vi "Read Sweep Configuration Example.vi"   [LabVIEW 2019, in "Sweep Control.lvclass"]
uses:
  Sweep Control.lvclass
  Typedefs/Enum - Experiments.ctl
  Typedefs/Continuous B Sweep JSON--Cluster.ctl
  Typedefs/Enum - Priority.ctl
  Typedefs/Enum - Action.ctl
  Typedefs/Cluster - ScanControl.ctl
  Typedefs/ScanControl.ctl
  Typedefs/Cluster - ScanParamters.ctl
  Typedefs/ScanParamters.ctl
  Typedefs/Sweep Control JSON--Cluster.ctl
  <userlib>/LevyLab/Transport/Transport/Typedefs/Lockin_Sweep JSON--Cluster.ctl
  <userlib>/LevyLab/Transport/Transport/Transport.lvclass
  <userlib>/LevyLab/Transport/Control Experiment/Typedefs/Wiring Description--cluster.ctl
  <userlib>/LevyLab/Transport/Control Experiment/Control Experiment.lvclass
  <userlib>/LevyLab/Transport/Control Experiment/Typedefs/Experiment Description--cluster.ctl
  <userlib>/LevyLab/Lockin-Multichannel/Instrument.DAQ/Typedefs/REF.Channel--Cluster--Array.ctl
  <userlib>/LevyLab/Lockin-Multichannel/Instrument.DAQ/Instrument.DAQ.lvclass
  <userlib>/LevyLab/Lockin-Multichannel/Instrument.DAQ/Typedefs/AO.Channel--Cluster--Array.ctl
  <userlib>/LevyLab/Transport/Control Experiment/Typedefs/Instruments--cluster.ctl
  <userlib>/LevyLab/Krohn Hite 7008/KH7008/typedefs/Filter--Enum.ctl
  <userlib>/LevyLab/Krohn Hite 7008/KH7008/KH7008.lvlib
  <userlib>/LevyLab/Krohn Hite 7008/KH7008/typedefs/couple--Enum.ctl
  <userlib>/LevyLab/Krohn Hite 7008/KH7008/typedefs/shunt--enum.ctl
  <userlib>/LevyLab/Krohn Hite 7008/KH7008/typedefs/Input--Enum.ctl
  <userlib>/LevyLab/Krohn Hite 7008/KH7008/typedefs/gain--enum.ctl
  <userlib>/LevyLab/Krohn Hite 7008/KH7008/typedefs/channel--numeric.ctl
  <userlib>/LevyLab/Krohn Hite 7008/KH7008/typedefs/channelProperties--Cluster.ctl
  <userlib>/LevyLab/Krohn Hite 7008/KH7008/typedefs/allChannelProperties--Array.ctl
  <userlib>/LevyLab/Lockin-Multichannel/Instrument.DAQ/Typedefs/AO.Channel.Function--Enum.ctl
  <userlib>/LevyLab/Lockin-Multichannel/Instrument.DAQ/Typedefs/AO.Channel--Cluster.ctl
  <userlib>/LevyLab/Lockin-Multichannel/Instrument.DAQ/Typedefs/REF.Channel--Cluster.ctl
  <userlib>/LevyLab/Transport/Control Experiment/Typedefs/Instrument Types--enum.ctl
panel:
  # "See block diagram for example of how to use ReadSweepConfigurationFile.vi"
types:
  T1 = typedef "Transport.lvclass/Lockin_Sweep JSON--Cluster.ctl" = cluster{"initialWaitTime":dbl, "sweepTime":dbl, "Return to Start":bool, "sweepChannels":cluster{"Enable?":bool, "Channel":u16, "Start":dbl, "End":dbl, "Pattern":enum16{"Ramp /", "Ramp /\\", "Smooth Ramp _/", "Smooth Ramp _/\\_", "Table"}, "Table":dbl[]}[], "sweepTables":cluster{"Ch":i32, "Table":dbl[]}[]}
  T2 = typedef "Sweep Control.lvclass/Sweep Control JSON--Cluster.ctl" = cluster{"Experiment":T3, "Repeat Experiment":i32, "Scan control":T4, "Scan parameters":T8}
  T3 = typedef "Sweep Control.lvclass/Enum - Experiments.ctl" = enum16{"LockinTime", "LockinSweep", "LockinDelayLine"}
  T4 = typedef "Sweep Control.lvclass/ScanControl.ctl" = T5[]
  T5 = typedef "Sweep Control.lvclass/Cluster - ScanControl.ctl" = cluster{"Priority":T6, "Scan name":T7}
  T6 = typedef "Sweep Control.lvclass/Enum - Priority.ctl" = enum16{"Priority 0", "Priority 1", "Priority 2", "Priority 3", "Priority 4", "Priority 5"}
  T7 = typedef "Sweep Control.lvclass/Enum - Action.ctl" = enum16{"OFF", "time", "Lockin Amplitude", "Lockin Frequency", "Lockin Bias", "Delay", "Strain", "DAQ Bias", "Magnet Field", "Temperature", "MW f1", "MW f2", "MW Amplitude1", "MW Amplitude2"}
  T8 = typedef "Sweep Control.lvclass/ScanParamters.ctl" = T9[]
  T9 = typedef "Sweep Control.lvclass/Cluster - ScanParamters.ctl" = cluster{"Start":dbl, "End":dbl, "Step":dbl, "Rate":dbl, "Waveform type":enum16{"linear", "triangle", "power"}, "wait (ms or K)":dbl, "Address":string, "channel":i32}
  T10 = typedef "Sweep Control.lvclass/Continuous B Sweep JSON--Cluster.ctl" = cluster{"Continuous B Sweep":cluster{"Experiment":T3, "B field values":dbl[]}, "Experiment Description":T11, "Wiring Configuration":T14, "Lockin":cluster{"AOconfig":T15, "REFconfig":T18}, "Krohn Hite":cluster{"Channel Setting":T20}}
  T11 = typedef "Control Experiment.lvclass/Experiment Description--cluster.ctl" = cluster{"User":string, "Device":string, "Device Path":path, "Device Description":string, "Experiment Path":path, "Experiment Description":string, "Instrument":string, "Instruments":T12[], "Sweep":cluster{"key":string, "value":variant}[]}
  T12 = typedef "Control Experiment.lvclass/Instruments--cluster.ctl" = cluster{"class path":path, "Address":string, "Type":T13}
  T13 = typedef "Control Experiment.lvclass/Instrument Types--enum.ctl" = enum16{"DAQ", "Amplifier", "Temperature", "Magnet", "Rotator", "Level", "Capacitance", "Delay Line", "Strain Cell", "VNA", "Source"}
  T14 = typedef "Control Experiment.lvclass/Wiring Description--cluster.ctl" = cluster{"Lockin Ch":i32[], "KH":cluster{"Electrodes":string[], "Labels":string[]}, "not KH":cluster{"Electrodes":string[], "Labels":string[]}}
  T15 = typedef "Instrument.Lockin.lvlib/Instrument.DAQ.lvclass/AO.Channel--Cluster--Array.ctl" = T16[]
  T16 = typedef "Instrument.Lockin.lvlib/Instrument.DAQ.lvclass/AO.Channel--Cluster.ctl" = cluster{"Enable?":bool, "Channel":i32, "Amplitude":dbl, "Offset":dbl, "Frequency":dbl, "Phase":dbl, "Function":T17, "Sweeping?":bool, "Limit AC":bool, "Limit DC?":bool, "Duty Cycle":bool}
  T17 = typedef "Instrument.Lockin.lvlib/Instrument.DAQ.lvclass/AO.Channel.Function--Enum.ctl" = enum16{"sine", "square", "triangle", "saw"}
  T18 = typedef "Instrument.Lockin.lvlib/Instrument.DAQ.lvclass/REF.Channel--Cluster--Array.ctl" = T19[]
  T19 = typedef "Instrument.Lockin.lvlib/Instrument.DAQ.lvclass/REF.Channel--Cluster.ctl" = cluster{"Enable?":bool, "Channel":i32, "Frequency":dbl, "Phase":dbl, "TC":dbl, "Roll-Off":i32}
  T20 = typedef "KH7008.lvlib/allChannelProperties--Array.ctl" = T21[]
  T21 = typedef "KH7008.lvlib/channelProperties--Cluster.ctl" = cluster{"channel":T22, "gain":T23, "input":T24, "shunt":T25, "couple":T26, "filter":T27}
  T22 = typedef "KH7008.lvlib/channel--numeric.ctl" = u16
  T23 = typedef "KH7008.lvlib/gain--enum.ctl" = enum16{"1", "10", "100", "1000"}
  T24 = typedef "KH7008.lvlib/Input--Enum.ctl" = enum16{"OFF", "SE+", "SE-", "DIFF"}
  T25 = typedef "KH7008.lvlib/shunt--enum.ctl" = enum16{"Open", "50", "500", "5k", "50k", "10M"}
  T26 = typedef "KH7008.lvlib/couple--Enum.ctl" = enum16{"AC", "DC"}
  T27 = typedef "KH7008.lvlib/Filter--Enum.ctl" = enum16{"OFF", "ON"}
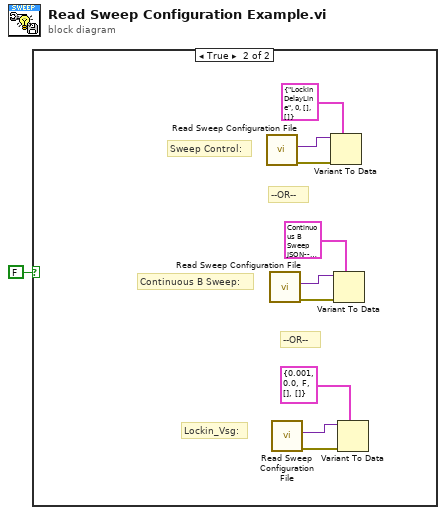
[diagram p0: block diagram]
diagram:
  n1 = case shown="True" FALSE {
    frame False {
    }
    frame True {
      # "Lockin_Vsg:"
      # "Continuous B Sweep:"
      # "Sweep Control:"
      # "--OR--"
      # "--OR--"
      n2 = call "Read Sweep Configuration File.vi"() -> ("error out"=w10:errorcluster, "Data"=w6:variant)  [unwired: 9 in, 1 out]
      n3 = call "Read Sweep Configuration File.vi"() -> ("error out"=w7:errorcluster, "Data"=w5:variant)  [unwired: 9 in, 1 out]
      n4 = call "Read Sweep Configuration File.vi"() -> ("error out"=w9:errorcluster, "Data"=w8:variant)  [unwired: 9 in, 1 out]
      n5 = Variant To Data(error in=w10, type=T2 {"Experiment"=enum."LockinDelayLine", "Repeat Experiment"=0, "Scan control"=[], "Scan parameters"=[]} ("SweepControl"), Variant=w6) -> ()  [unwired: 2 out]
      n6 = Variant To Data(error in=w7, type=T10 {"Continuous B Sweep"={"Experiment"=enum."LockinDelayLine", "B field values"=[]}, "Experiment Description"={"User"="", "Device"="", "Device Path"=path "", "Device Description"="", "Experiment Path"=path "", "Experiment Description"="", "Instrument"="", "Instruments"=[], "Sweep"=[]}, "Wiring Configuration"={"Lockin Ch"=[], "KH"={"Electrodes"=[], "Labels"=[]}, "not KH"={"Electrodes"=[], "Labels"=[]}}, "Lockin"={"AOconfig"=[], "REFconfig"=[]}, "Krohn Hite"={"Channel Setting"=[]}} ("ContinuousBSweep"), Variant=w5) -> ()  [unwired: 2 out]
      n7 = Variant To Data(error in=w9, type=T1 {"initialWaitTime"=0.001, "sweepTime"=0.0, "Return to Start"=FALSE, "sweepChannels"=[], "sweepTables"=[]} ("LockinVsg Sweep"), Variant=w8) -> ()  [unwired: 2 out]
    }
  }
